vi "getEvents.vi"(8 "error in (no error)":errorcluster, 11 "SettingsEventsManager in":refnum<class "SettingsEventsManager.lvclass">) -> (0 "error out":errorcluster, 2 "settingsEvents":T1, 3 "SettingsEventsManager out":refnum<class "SettingsEventsManager.lvclass">)   [LabVIEW 2009, in "Tools.lvlib" / "Settings.lvlib" / "SettingsEventsManager.lvclass"]
uses:
  SettingsEventsManager.lvclass
  SettingsEventsManager.lvclass/SettingsEventsManager.ctl
  Settings.lvlib
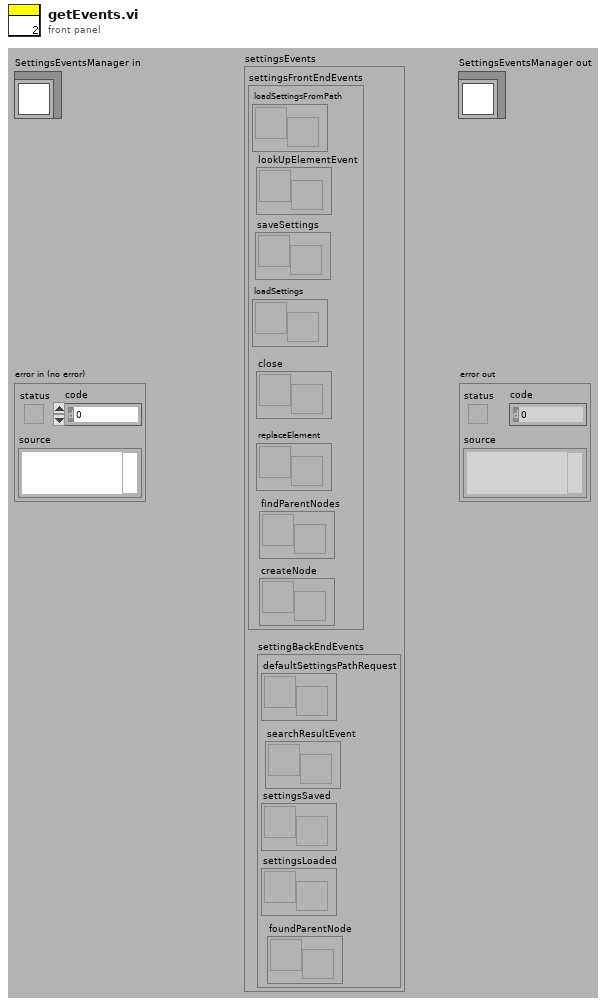
[diagram p1: front panel]
types:
  T1 = cluster{"settingsFrontEndEvents":cluster{"loadSettingsFromPath":refnum<user-event>, "lookUpElementEvent":refnum<user-event>, "saveSettings":refnum<user-event>, "loadSettings":refnum<user-event>, "close":refnum<user-event>, "replaceElement":refnum<user-event>, "findParentNodes":refnum<user-event>, "createNode":refnum<user-event>}, "settingBackEndEvents":cluster{"defaultSettingsPathRequest":refnum<user-event>, "searchResultEvent":refnum<user-event>, "settingsSaved":refnum<user-event>, "settingsLoaded":refnum<user-event>, "foundParentNode":refnum<user-event>}}
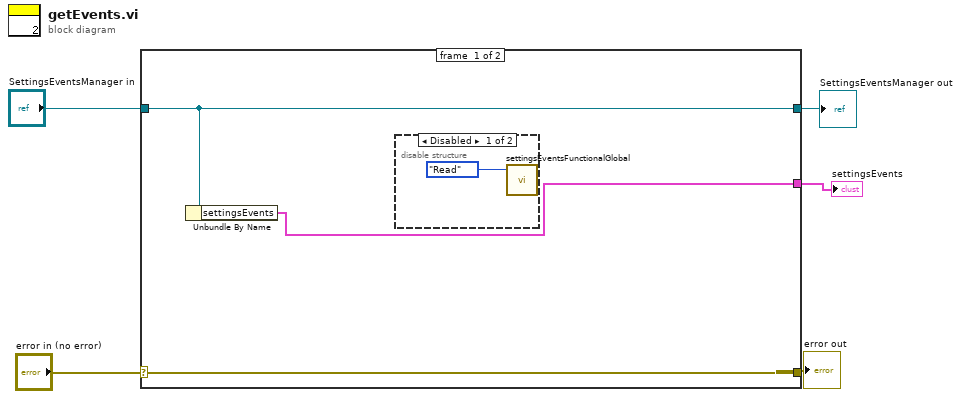
[diagram p0: block diagram]
diagram:
  n1 = case shown="No Error" "error in (no error)" {
    selector: "error in (no error)" -> [w8 w11]
    tunnel: [w8 w11] -> w4
    tunnel: [w7 w10] -> w2
    tunnel: "SettingsEventsManager in" -> [w7 w10]
    tunnel: [w6 _] -> w1
    frame #0 {
      n2 = Unbundle By Name(w7) -> ("settingsEvents"=w6:T1)
      n3 = disable-structure shown="Disabled" {
        frame #0 {
          n4 = call "settingsEventsFunctionalGlobal.vi"("Action"=enum16{"Write", "Read"}."Read") -> ()  [unwired: 10 in, 1 out]
        }
        frame #1 {
        }
      }
    }
    frame #1 {
    }
  }
  "error out" <- w4
  "SettingsEventsManager out" <- w2
  "settingsEvents" <- w1
